vi "globalTearDown.vi"(8 "error in":errorcluster, 11 "Deployment in":refnum<class "Deployment.lvclass">) -> (0 "error out":errorcluster, 3 "Deployment out":refnum<class "Deployment.lvclass">)   [LabVIEW 2020, in "Deployment.lvclass"]
uses:
  Deployment.lvclass
  Deployment.lvclass/Deployment.ctl
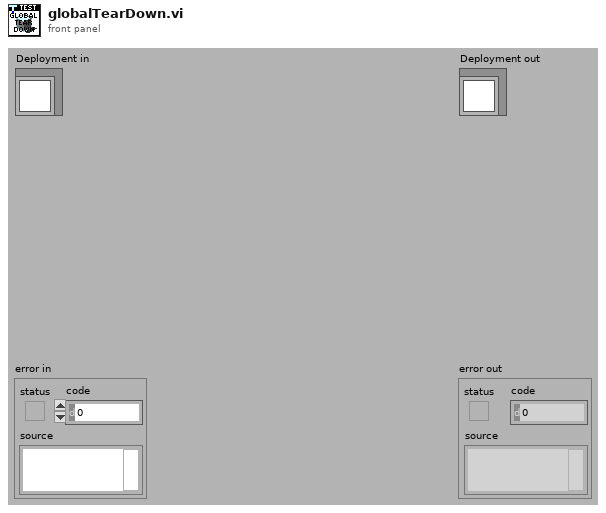
[diagram p1: front panel]
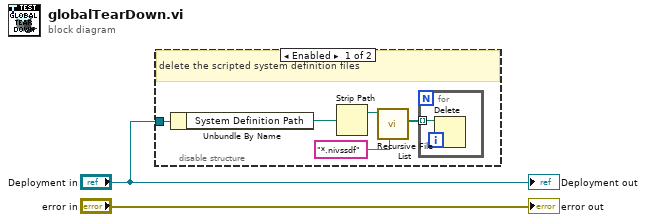
[diagram p0: block diagram]
diagram:
  n1 = disable-structure shown="Enabled" {
    disable-tunnel: "Deployment in" -> [w7 _]
    frame Enabled {
      # "delete the scripted system definition files"
      n2 = Unbundle By Name(w7) -> ("System Definition Path"=w4:path)
      n3 = Strip Path(path=w4) -> (stripped path=w3:path)  [unwired: 1 out]
      n4 = call <vilib>:"Recursive File List.vi"("pattern"="*.nivssdf", "Folder Path"=w3) -> ("All Files in Dir"=w5:path[])  [unwired: 5 in, 4 out]
      n5 = for {
        tunnel: w5 -> [w8] mode=indexing
        n6 = Delete(path (use dialog)=w8) -> ()  [unwired: 4 in, 3 out]
      }
    }
    frame Disabled {
    }
  }
  "error out" <- "error in"
  "Deployment out" <- "Deployment in"
